vi "Apply Configuration.vi"(8 "error in":errorcluster, 11 "Scope Base in":refnum<class "Scope Base.lvclass">) -> (0 "error out":errorcluster, 3 "Scope Base out":refnum<class "Scope Base.lvclass">)   [LabVIEW 2023, in "Scope Base.lvlib" / "Scope Base.lvclass"]
uses:
  Scope Base.lvclass
  Scope Base.lvclass/Scope Base.ctl
  Interfaces/IConfigure/IConfigure.lvclass
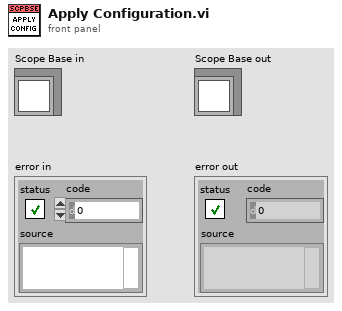
[diagram p1: front panel]
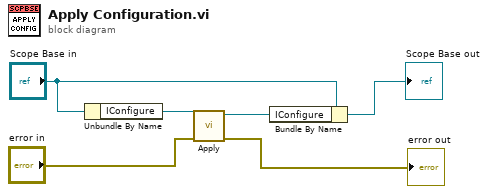
[diagram p0: block diagram]
diagram:
  n1 = Unbundle By Name("Scope Base in") -> ("IConfigure"=w5:refnum<class "IConfigure.lvclass">)
  n2 = call-dynamic "Apply.vi"("Error In"="error in", "IConfigure in"=w5) -> ("Error Out"=→"error out":errorcluster, "IConfigure out"=w1:refnum<class "IConfigure.lvclass">)  [unwired: 8 in]
  n3 = Bundle By Name(cluster="Scope Base in", "IConfigure"=w1) -> (→"Scope Base out":refnum<class "Scope Base.lvclass">)
